vi "Check Repeat.vi"(11 "Array":i64[](array[numeric])) -> (2 "Repeat?":bool, 3 "Pattern Length":i32)   [LabVIEW 2021]
uses:
  b14f3743-932c-41a9-b51e-8efdce2b83f2.vi
  <vilib>/Comparison/Equal/Equal Functor/Equal Functor.lvclass
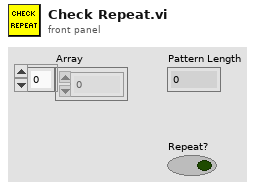
[diagram p1: front panel]
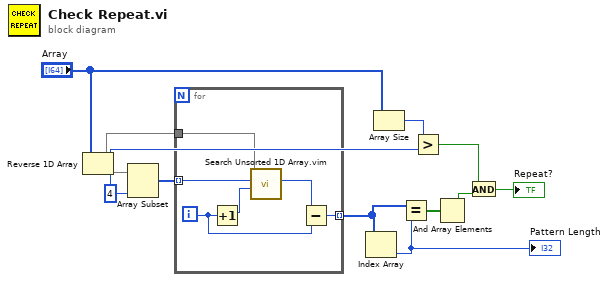
[diagram p0: block diagram]
diagram:
  w6 = 4
  n1 = Reverse 1D Array(array="Array") -> (reversed array=w2:i64[])
  n2 = Array Subset(array=w2, length=w6) -> (w1:i64[])  [unwired: 1 in]
  n3 = for {
    tunnel: w1 -> [w16] mode=indexing
    tunnel: w2 -> [w17]
    tunnel: [w12] -> w3 mode=indexing
    i -> [w14]
    n4 = Increment(x=w14) -> (x+1=w15:i32)
    n5 = call "Search Unsorted 1D Array.vim"("start index (0)"=w15, "element"=w16, "unsorted 1D array"=w17) -> ("index of element"=w13:i32)  [unwired: 8 in]
    n6 = Subtract(x=w13, y=w14) -> (x-y=w12:i32)
  }
  n7 = Index Array(array=w3) -> (element=w11:i32)  [unwired: 1 in]
  "Pattern Length" <- w11
  n8 = Array Size(array="Array") -> (size(s)=w5:i32)
  n9 = Equal?(x=w3, y=w11) -> (x = y?=w4:bool[])
  n10 = Greater?(x=w5, y=w6) -> (0:w8:bool)
  n11 = And Array Elements(Boolean array=w4) -> (logical AND=w7:bool)
  n12 = And(x=w8, y=w7) -> (x .and. y?=→"Repeat?":bool)
